vi "linear interp iiii- complex.vi"(0 "z":cdb[](array[numeric]), 11 "center":i32=-1) -> (3 "directed sigma - abs":dbl, 4 "left":cdb, 6 "center":cdb, 8 "right":cdb, 10 "directed sigma":cdb, 12 "intercept":cdb, 13 "slope":cdb)   [LabVIEW 2020]
uses:
  <vilib>/Analysis/baseanly.llb/Complex A x B.vi
  Q - not nan -- real.vi
  <vilib>/Analysis/Matrix/Numeric/Conversions/Array To Matrix.vi
  <vilib>/Analysis/Matrix/Numeric/Conversions/Array To Matrix - RA2.vi
  <vilib>/Analysis/baseanly.llb/Inverse Matrix.vi
  <vilib>/Analysis/baseanly.llb/Real Inverse Matrix.vi
  <vilib>/Analysis/NI_AALBase.lvlib
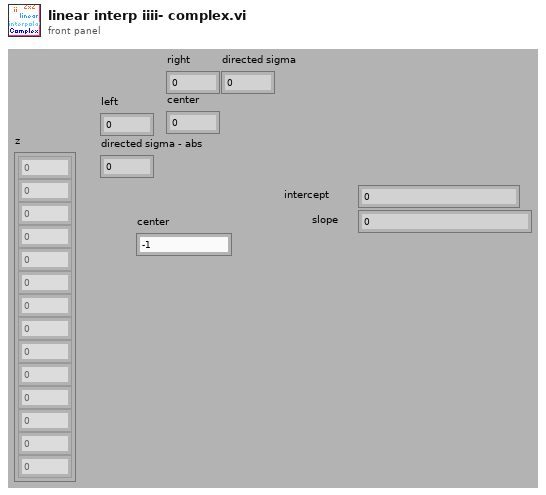
[diagram p1: front panel]
types:
  T1 = typedef "NI_Matrix.lvlib/RealMatrix.ctl" = dbl[][]
  T2 = typedef "NI_Matrix.lvlib/ComplexMatrix.ctl" = cdb[][]
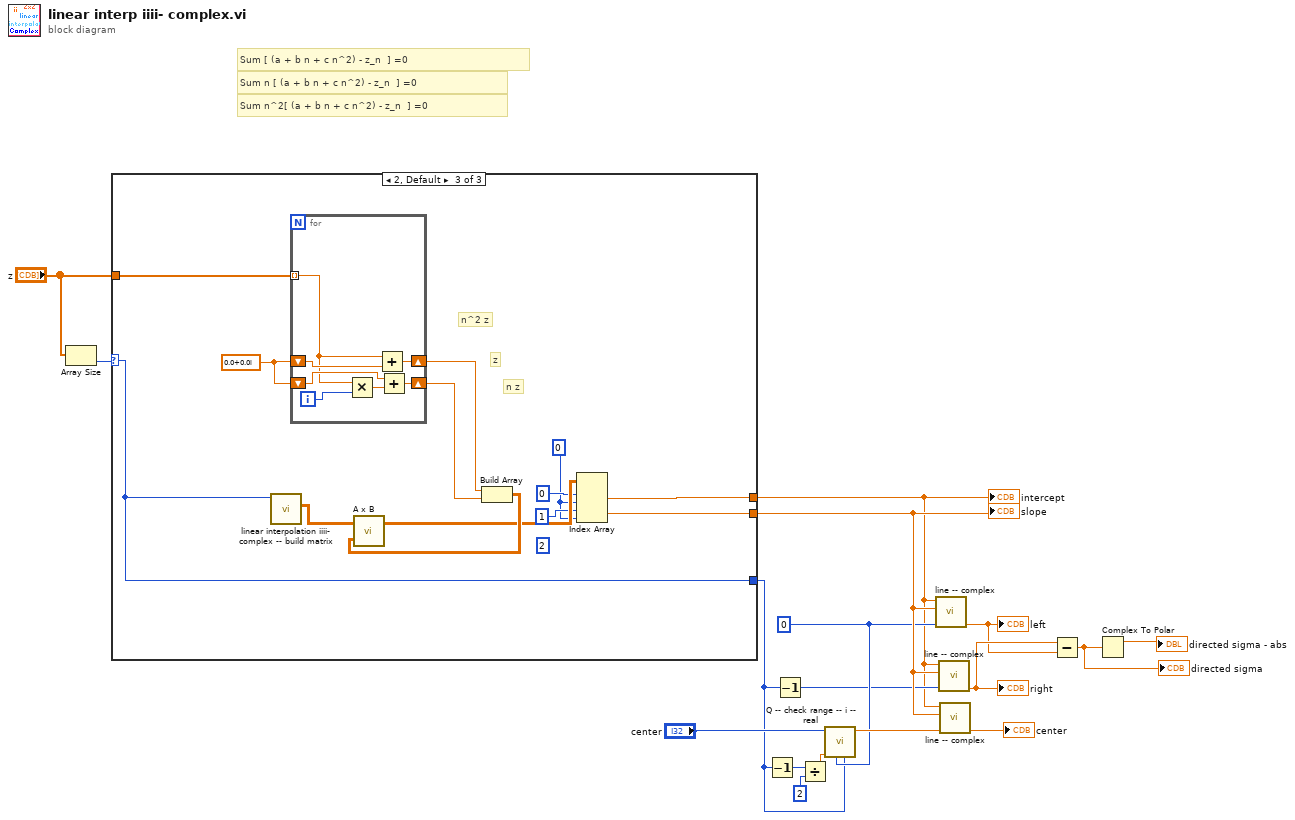
[diagram p0: block diagram]
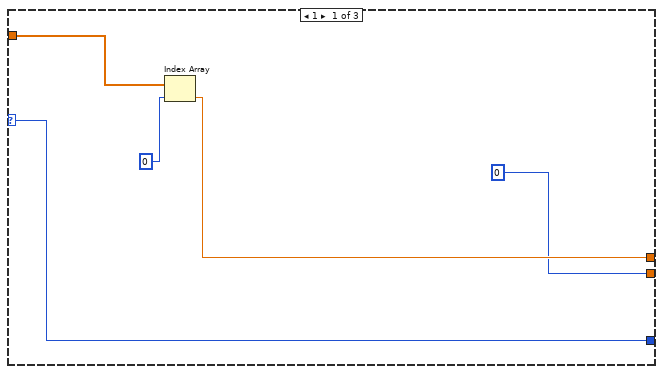
[diagram p2: hidden frame]
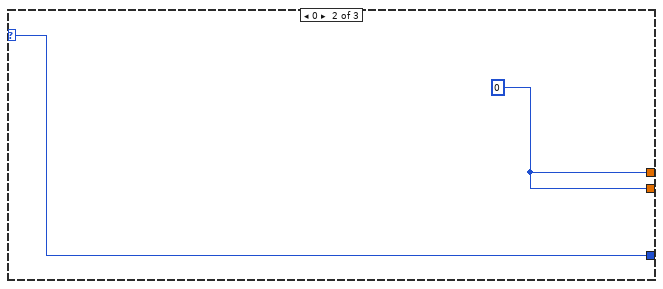
[diagram p3: hidden frame]
diagram:
  w9 = 0 ("n")
  # "Sum n^2[ (a + b n + c n^2) - z_n  ] =0"
  # "Sum n [ (a + b n + c n^2) - z_n  ] =0"
  # "Sum [ (a + b n + c n^2) - z_n  ] =0"
  n1 = Array Size(array="z") -> (size(s)=w1:i32)
  n2 = case shown="2, Default" w1 {
    selector: w1 -> [w19 w24 w25]
    tunnel: [w20 w23 w27] -> w3
    tunnel: [0 ("index") w23 w26] -> w10
    tunnel: "z" -> [w22 _ w37]
    tunnel: [w19 w24 w25] -> w7
    frame 1 {
      n3 = Index Array(array=w22, index=0) -> (element=w20:cdb)
    }
    frame 0 {
      w23 = 0 ("index")
    }
    frame 2, Default {
      (unwired) 2 ("index (row)")
      w28 = 0 ("index (row)")
      w36 = cdb 0.0+0.0i
      # "n z"
      # "z"
      # "n^2 z"
      n4 = call "linear interpolation iiii- complex -- build matrix.vi"("N"=w25) -> ("Inverse Matrix"=w33:T1)  [unwired: 10 in]
      n5 = for {
        tunnel: w37 -> [w38] mode=indexing
        shift-right: [w44] -> w35
        shift-left: w36 -> [w43]
        shift-right: [w41] -> w34
        shift-left: w36 -> [w40]
        i -> [w39]
        n6 = Multiply(x=w38, y=w39) -> (x*y=w42:cdb)
        n7 = Add(x=w38, y=w43) -> (x+y=w44:cdb)
        n8 = Add(x=w40, y=w42) -> (x+y=w41:cdb)
      }
      n9 = Build Array(w35, w34) -> (w32:T2)
      n10 = call-poly <vilib>:"A x B.vi"("B"=w32, "A"=w33) -> ("A x B"=w31:T2)  [unwired: 1 out]
      n11 = Index Array(array=w31, index (row) #1=0 ("index (row)"), index (col) #1=w28, index (row) #2=1 ("index (row)"), index (col) #2=w28) -> (element #1=w27:cdb, element #2=w26:cdb)
    }
  }
  "slope" <- w10
  "intercept" <- w3
  n12 = Decrement(x=w7) -> (x-1=w17:i32)
  n13 = Decrement(x=w7) -> (x-1=w6:i32)
  n14 = Divide(x=w17, y=2 ("n")) -> (x/y=w8:dbl)
  n15 = call "Q -- check range -- i -- real.vi"("upper"=w7, "lower"=w9, "default"=w8, "number"="center") -> ("number in range"=w14:dbl)  [unwired: 5 in, 2 out]
  n16 = call "line -- complex.vi"("n"=w9, "slope"=w10, "intercept"=w3) -> ("value"=w11:cdb)  [unwired: 7 in, 1 out]
  "left" <- w11
  n17 = call "line -- complex.vi"("n"=w6, "slope"=w10, "intercept"=w3) -> ("value"=w12:cdb)  [unwired: 7 in, 1 out]
  "right" <- w12
  n18 = call "line -- complex.vi"("n"=w14, "slope"=w10, "intercept"=w3) -> ("value"=→"center":cdb)  [unwired: 7 in, 1 out]
  n19 = Subtract(x=w12, y=w11) -> (x-y=w4:cdb)
  "directed sigma" <- w4
  n20 = Complex To Polar(r * e^(i*theta)=w4) -> (r=→"directed sigma - abs":dbl)  [unwired: 1 out]
